vi "Analyse Data.vi"(8 "error in (no error)":errorcluster, 11 "Data In":dbl[](array[numeric])) -> (0 "error out":errorcluster)   [LabVIEW 2023]
uses:
  <vilib>/Analysis/baseanly.llb/Mean (DBL).vi
  <vilib>/Analysis/NI_AALBase.lvlib
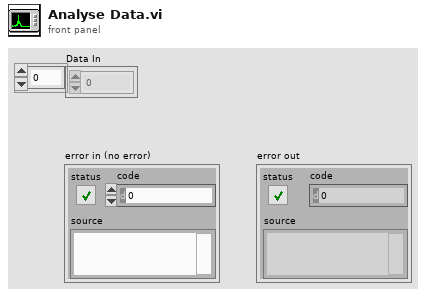
[diagram p1: front panel]
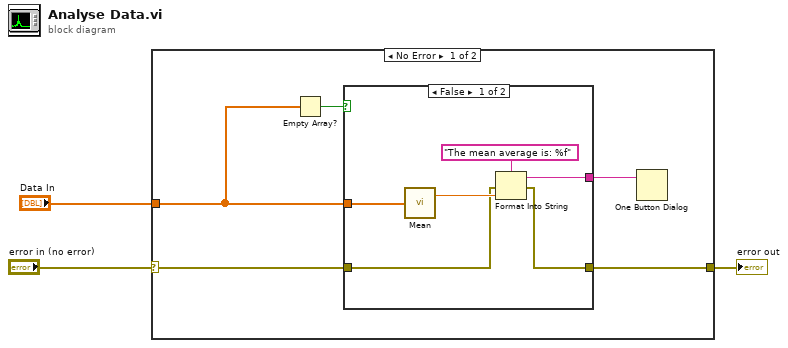
[diagram p0: block diagram]
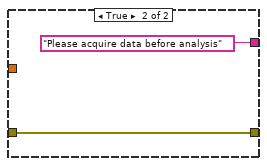
[diagram p2: hidden frame]
diagram:
  n1 = case shown="No Error" "error in (no error)" {
    selector: "error in (no error)" -> [w5 w17]
    tunnel: [w4 w17] -> w2
    tunnel: "Data In" -> [w6 _]
    frame No Error {
      n2 = Empty Array?(array=w6) -> (empty?=w8:bool)
      n3 = case shown="False" w8 {
        tunnel: [w11 "Please acquire data before analysis"] -> w7
        tunnel: w6 -> [w14 _]
        tunnel: w5 -> [w10 w15]
        tunnel: [w9 w15] -> w4
        frame False {
          n4 = call-poly <vilib>:"Mean.vi"("X"=w14) -> ("mean"=w12:dbl)  [unwired: 1 out]
          n5 = Format Into String(format string="The mean average is: %f", error in=w10, w12) -> (resulting string=w11:string, error out=w9:errorcluster)  [unwired: 1 in]
        }
        frame True {
        }
      }
      n6 = One Button Dialog(message=w7) -> ()  [unwired: 1 in, 1 out]
    }
    frame Error {
    }
  }
  "error out" <- w2
